vi "Quit message scheduler.vi"(11 "RT Queues":T1) -> (3 "RT Queues out":T1)   [LabVIEW 2018, in "Message scheduler.lvlib"]
uses:
  Message scheduler.lvlib
  Type Defs/scheduled message cluster.ctl
  Type Defs/Queues cluster.ctl
  ICL-LabVIEW_General/Message Scheduler/message scheduler.lvclass
types:
  T1 = typedef "Queues cluster.ctl" = cluster{"RT Message":refnum<queue>, "RT Comms":refnum<queue>, "RT Data":refnum<queue>, "RT FIFO":refnum<queue>, "message scheduler":refnum<class "message scheduler.lvclass">}
  T2 = typedef "Message scheduler.lvlib/scheduled message cluster.ctl" = cluster{"message element":cluster{"Message":string, "Data":variant}, "schedule":cluster{"Repeats":i16, "Period (ms)":u32, "ID":u32, "Queue":enum16{"Message", "Comms"}, "T0":u32}, "Action":enum16{"New", "Remove", "Quit"}}
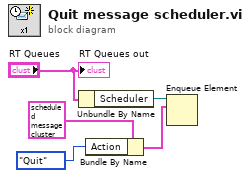
[diagram p0: block diagram]
diagram:
  n1 = Unbundle By Name("RT Queues") -> ("Scheduler"=w4:refnum<queue>)
  n2 = Bundle By Name(cluster=T2 {"message element"={"Message"="", "Data"=variant}, "schedule"={"Repeats"=0, "Period (ms)"=0, "ID"=0, "Queue"=enum."Message", "T0"=0}, "Action"=enum."New"} ("Scheduled message"), "Action"=enum16{"New", "Remove", "Quit"}."Quit") -> (w2:T2)
  n3 = Enqueue Element(queue=w4, element=w2) -> ()  [unwired: 2 in, 3 out]
  "RT Queues out" <- "RT Queues"
